vi "time.vi"() -> ()   [LabVIEW 2014]
panel:
  in  "stop":bool
  in  "Led sequence":bool
  out "Led3":bool
  out "Led2":bool
  out "Led1":bool
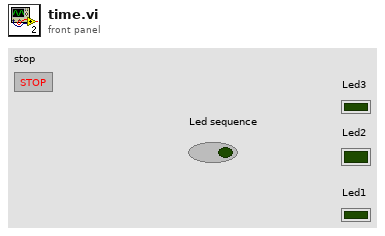
[diagram p1: front panel]
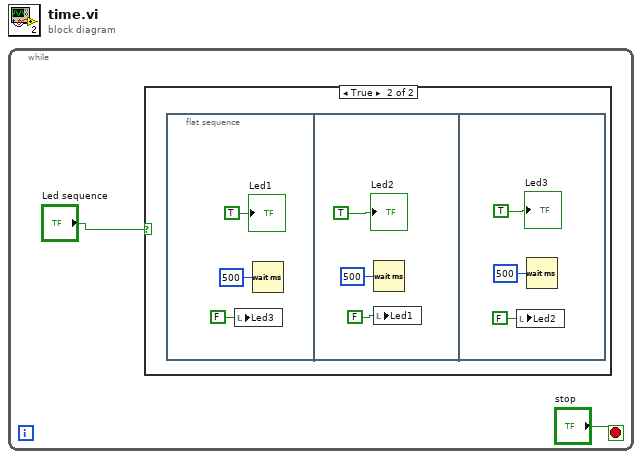
[diagram p0: block diagram]
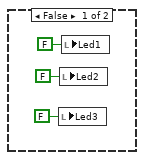
[diagram p2: hidden frame]
diagram:
  n1 = while {
    stop <- "stop" stop-if-true
    n2 = case shown="True" "Led sequence" {
      frame False {
        n3 = local write "Led3"(FALSE ("Led3")) -> ()
        n4 = local write "Led2"(FALSE ("Led2")) -> ()
        n5 = local write "Led1"(FALSE ("Led1")) -> ()
      }
      frame True {
        n6 = flat-sequence {
          frame #0 {
            n7 = local write "Led3"(FALSE ("Led3")) -> ()
            n8 = Wait (ms)(milliseconds to wait=u32 500) -> ()  [unwired: 1 out]
            "Led1" <- TRUE ("Led1")
          }
          frame #1 {
            n9 = Wait (ms)(milliseconds to wait=u32 500) -> ()  [unwired: 1 out]
            n10 = local write "Led1"(FALSE ("Led1")) -> ()
            "Led2" <- TRUE ("Led2")
          }
          frame #2 {
            n11 = local write "Led2"(FALSE ("Led2")) -> ()
            n12 = Wait (ms)(milliseconds to wait=u32 500) -> ()  [unwired: 1 out]
            "Led3" <- TRUE ("Led3")
          }
        }
      }
    }
  }
